vi "broadcastReg-TestCore.vi"(7 "status":string="status@source >> api@target -><register>\nstatus@source >> api2@target -><register>", 9 "Target":string="target", 10 "Source":string="source", 11 "Status":string="status") -> (3 "Response Message Info":string[](array[string]))   [LabVIEW 2017]
uses:
  user.lib/_NEVSTOP/Communicable State Machine(CSM)/_Support/Common/Trim Single line Text.vi
  user.lib/_NEVSTOP/Communicable State Machine(CSM)/_Support/BroadcastRegistry/BroadcastRegistry.lvclass
  user.lib/_NEVSTOP/Communicable State Machine(CSM)/Communicable State Machine.lvlib
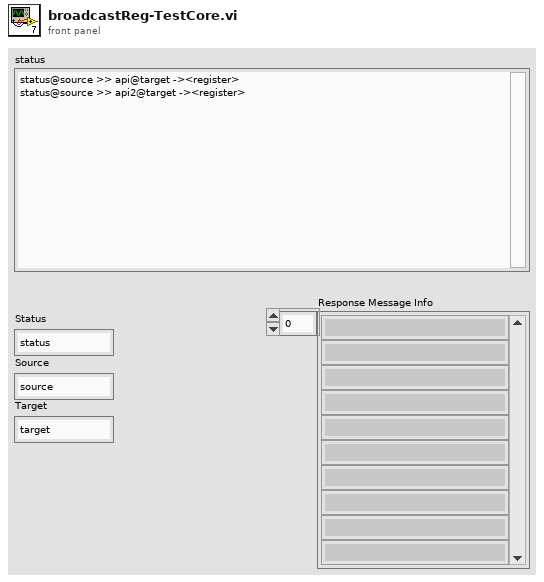
[diagram p1: front panel]
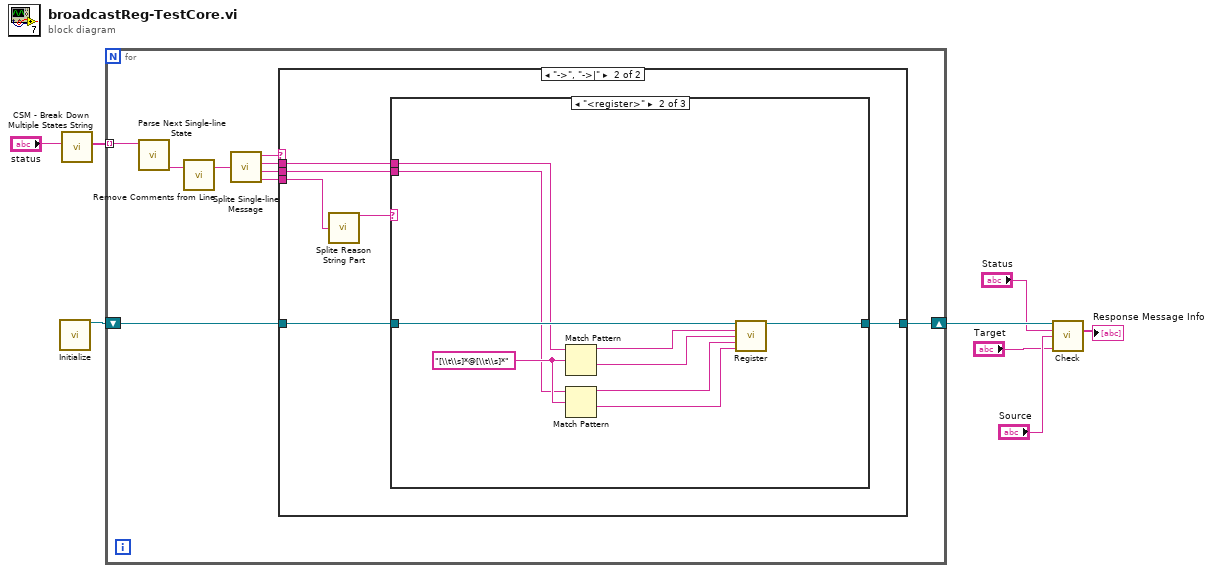
[diagram p0: block diagram]
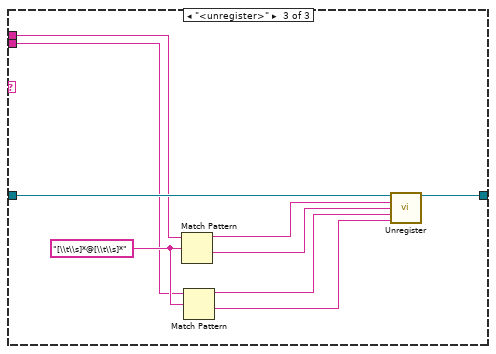
[diagram p4: hidden frame]
diagram:
  n1 = call "Initialize.vi"() -> ("BroadcastRegistry out"=w6:refnum<class "BroadcastRegistry.lvclass">)  [unwired: 15 in]
  n2 = call "CSM - Break Down Multiple States String.vi"("States"="status") -> ("Multiple States"=w7:string[])  [unwired: 10 in]
  n3 = for {
    tunnel: w7 -> [w15] mode=indexing
    shift-right: [w9] -> w5
    shift-left: w6 -> [w10]
    n4 = call "Parse Next Single-line State.vi"("States Queue"=w15) -> ("Next Single-line State"=w16:string)  [unwired: 9 in, 1 out]
    n5 = call "Remove Comments from Line.vi"("single-line text"=w16) -> ("single-line text without comments"=w17:string)  [unwired: 2 in]
    n6 = call "Splite Single-line Message.vi"("single-line text"=w17) -> ("operator"=w14:string, "state"=w13:string, "args"=w12:string, "source/target"=w11:string)  [unwired: 6 in]
    n7 = case shown="\"->\", \"->|\"" w14 {
      tunnel: w13 -> [_ w24]
      tunnel: w12 -> [_ w23]
      tunnel: w11 -> [_ w20]
      tunnel: w10 -> [w18 w22]
      tunnel: [w18 w21] -> w9
      frame "False", Default {
      }
      frame "->", "->|" {
        n8 = call "Splite Reason String Part.vi"("Single-line -& Reason"=w20) -> ("CSM Name"=w19:string)  [unwired: 12 in, 2 out]
        n9 = case shown="\"<register>\"" w19 {
          tunnel: w24 -> [_ w31 w40]
          tunnel: w23 -> [_ w30 w39]
          tunnel: w22 -> [w25 w34 w43]
          tunnel: [w25 w33 w42] -> w21
          frame "False", Default {
          }
          frame "<register>" {
            w32 = "[\\t\\s]*@[\\t\\s]*" ("regular expression")
            n10 = Match Pattern(string=w31, regular expression=w32) -> (before substring=w26:string, after substring=w27:string)  [unwired: 1 in, 2 out]
            n11 = Match Pattern(string=w30, regular expression=w32) -> (before substring=w28:string, after substring=w29:string)  [unwired: 1 in, 2 out]
            n12 = call "Register.vi"("BroadcastRegistry in"=w34, "status"=w26, "source"=w27, "api"=w28, "target"=w29) -> ("BroadcastRegistry out"=w33:refnum<class "BroadcastRegistry.lvclass">)  [unwired: 10 in]
          }
          frame "<unregister>" {
            w41 = "[\\t\\s]*@[\\t\\s]*" ("regular expression")
            n13 = Match Pattern(string=w40, regular expression=w41) -> (before substring=w36:string, after substring=w37:string)  [unwired: 1 in, 2 out]
            n14 = Match Pattern(string=w39, regular expression=w41) -> (before substring=w35:string, after substring=w38:string)  [unwired: 1 in, 2 out]
            n15 = call "Unregister.vi"("BroadcastRegistry in"=w43, "Status"=w36, "Source"=w37, "api"=w35, "Target"=w38) -> ("BroadcastRegistry out"=w42:refnum<class "BroadcastRegistry.lvclass">)  [unwired: 10 in]
          }
        }
      }
    }
  }
  n16 = call "Check.vi"("BroadcastRegistry in"=w5, "Status"="Status", "Source"="Source", "Target"="Target") -> ("Response Message Info"=→"Response Message Info":string[])  [unwired: 10 in, 1 out]
